vi "Loop Async.vi"(10 "ExecAnchor":refnum<class "ExecAnchor.lvclass">, 11 "BluelinesRedlines in":refnum<class "BluelinesRedlines.lvclass">) -> ()   [LabVIEW 2020, in "VolatusGUIElements.lvlib" / "BluelinesRedlines.lvclass"]
uses:
  BluelinesRedlines.lvclass
  lv-exec-anchor/ExecAnchor/ExecAnchor.lvclass
  BluelinesRedlines.lvclass/BluelinesRedlines.ctl
  lv-exec-anchor/ExecAnchor/ExecAnchor.lvclass/ExecAnchor.ctl
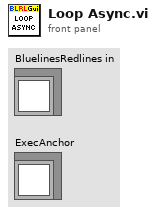
[diagram p1: front panel]
types:
  T1 = typedef "VolatusGUIElements.lvlib/BluelinesRedlines.lvclass/BLRL Control.ctl" = cluster{"Blue Lines":cluster{"Channel":string, "Low":string, "Value":dbl, "High":string, "Color":u32, "Remove Channel":bool}[], "Red Lines":cluster{"Channel":string, "Low":string, "Value":dbl, "High":string, "Color":u32, "Remove Channel":bool}[], "Import":bool, "Export":bool, "Blueline Status":bool, "Redlines Status":bool, "Group":string, "New Group":bool, "Dup Group":bool, "Remove Group":bool, "Add Blue Channel":bool, "Add Red Channel":bool, "Reset Redlines":bool}
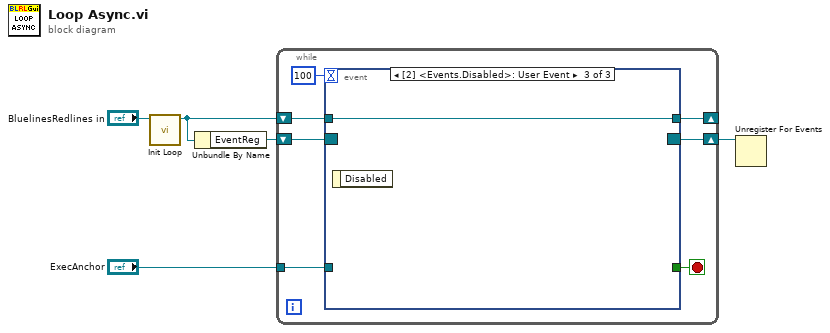
[diagram p0: block diagram]
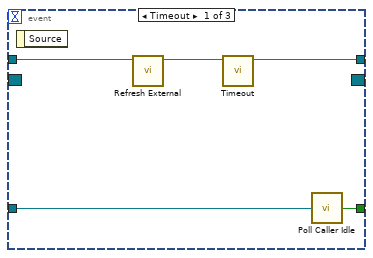
[diagram p2: hidden frame]
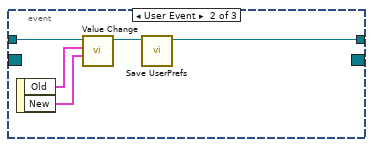
[diagram p3: hidden frame]
diagram:
  n1 = call "Init Loop.vi"("BluelinesRedlines in"="BluelinesRedlines in") -> ("BluelinesRedlines out"=w1:refnum<class "BluelinesRedlines.lvclass">)  [unwired: 9 in, 1 out]
  n2 = Unbundle By Name(w1) -> ("EventReg"=w4:refnum<event-registration>)
  n3 = while {
    shift-right: [w8] -> _
    shift-left: w1 -> [w10]
    shift-right: [w9] -> w3
    shift-left: w4 -> [w11]
    tunnel: "ExecAnchor" -> [w7]
    stop <- w6 stop-if-true
    n4 = event shown="[2] <Events.Disabled>: User Event" {
      selector: w11 -> [_ _ _]
      dyn-events: [_ _ _] -> w9
      timeout: 100 -> [_ _ _]
      tunnel: w10 -> [w14 w22 w23]
      tunnel: [w15 w18 w23] -> w8
      tunnel: w7 -> [w17 _ _]
      tunnel: [w16 _ _] -> w6
      event Timeout {
        n5 = event-data() -> ()  [unwired: 1 in, 1 out]
        n6 = call "Refresh External.vi"("BluelinesRedlines in"=w14) -> ("BluelinesRedlines out"=w13:refnum<class "BluelinesRedlines.lvclass">)  [unwired: 9 in, 1 out]
        n7 = call "Timeout.vi"("BluelinesRedlines in"=w13) -> ("BluelinesRedlines out"=w15:refnum<class "BluelinesRedlines.lvclass">)  [unwired: 9 in, 1 out]
        n8 = call "Poll Caller Idle.vi"("ExecAnchor in"=w17) -> ("Caller Idle"=w16:bool)  [unwired: 3 in, 1 out]
      }
      event User Event {
        n9 = event-data() -> ("Old"=w21:T1, "New"=w20:T1)  [unwired: 1 in]
        n10 = call "Value Change.vi"("New"=w20, "Old"=w21, "BluelinesRedlines in"=w22) -> ("BluelinesRedlines out"=w19:refnum<class "BluelinesRedlines.lvclass">)  [unwired: 7 in, 1 out]
        n11 = call "Save UserPrefs.vi"("BluelinesRedlines in"=w19) -> ("BluelinesRedlines out"=w18:refnum<class "BluelinesRedlines.lvclass">)  [unwired: 9 in, 1 out]
      }
      event User Event {
        n12 = event-data() -> ()  [unwired: 1 in, 1 out]
      }
    }
  }
  n13 = Unregister For Events(event registration refnum=w3) -> ()  [unwired: 1 in, 1 out]
